vi "Check and Get Scalar.vi"(8 "error in (no error)":errorcluster, 9 "test commands":string[](array[string]), 10 "variable name":string, 11 "pipe in":T1) -> (0 "error out":errorcluster, 1 "variable":string, 2 "all tests OK?":bool, 3 "pipe out":T1)   [LabVIEW 2013, in "GOLPI library.lvlib"]
doc: "Checks scalar variable and gets it from GNU Octave in one write-read cycle. 'variable name' is the name of the variable. 'test commands' is array of GNU Octave commands with boolean output applied to the variable. I.e. to read noncomplex double scalar variable 'x', following array should be supplied:\nisnumeric\nisscalar\n~isscomplex\nTests performed are:\nisnumeric(x)\nisscalar(x)\n~iscomplex(x)\nIf output of all tests is '1', output 'all tests OK?' is true."
uses:
  GOLPI library.lvlib
  LV Process.lvlibp/Pipe Handle.ctl
  Utilities/Custom Error Codes Enum Type Def.vi
  Globals.vi
  LV Process.lvlibp
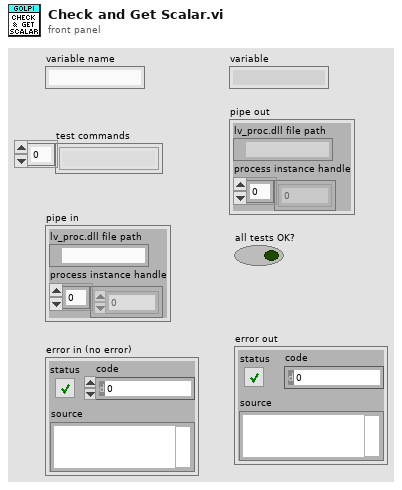
[diagram p1: front panel]
types:
  T1 = typedef "LV Process.lvlibp/Pipe Handle.ctl" = cluster{"lv_proc.dll file path":path, "process instance handle":u32[]}
  T2 = typedef "GOLPI library.lvlib/Custom Error Codes Enum Type Def.vi" = enum16{"no error", "00 working directory PAR1 missing", "01 octave binary PAR1 missing", "02 octave report error PAR1", "03 empty output last cmd PAR1", "04 missing temporary file PAR1", "10 var PAR1 not string", "11 var PAR1 not num, scal, ~compl", "12 var PAR1 not num, scal, compl", "13 var PAR1 not num, vect, ~compl", "14 var PAR1 not num, vect, compl", "15 var PAR1 not num, mat, ~compl", "16 var PAR1 not num, mat, ~compl", "99 not finished"}
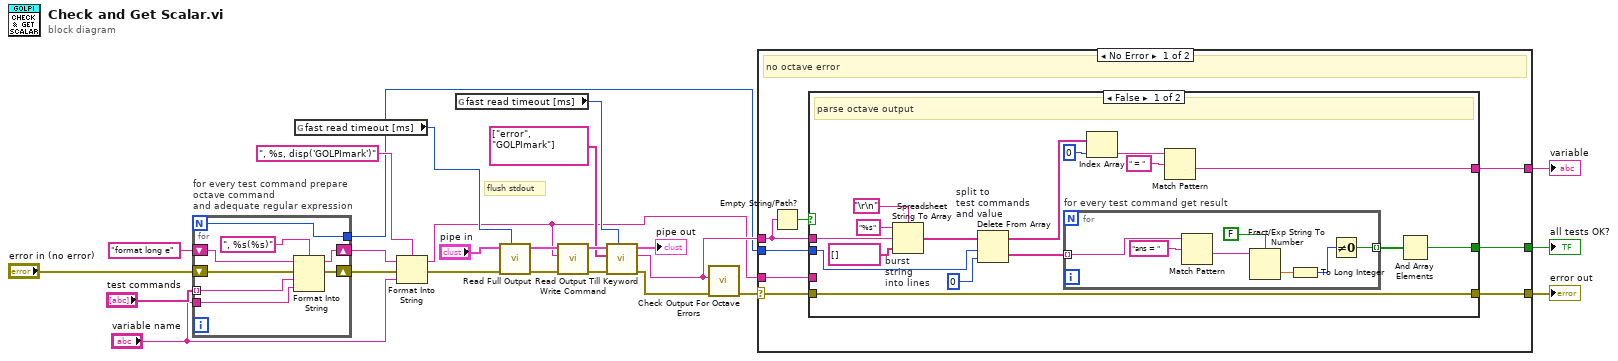
[diagram p0: block diagram]
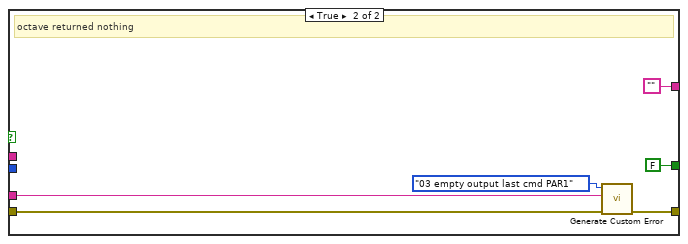
[diagram p2: hidden frame]
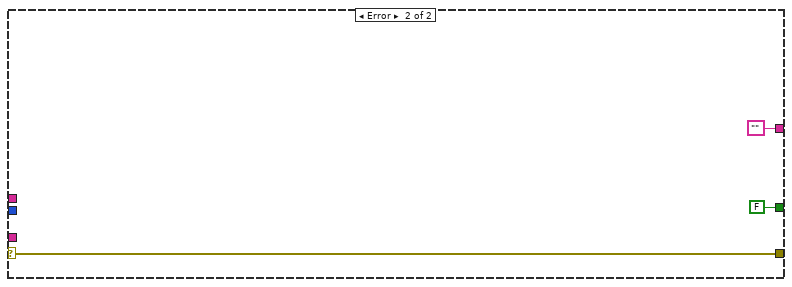
[diagram p3: hidden frame]
diagram:
  # "flush stdout"
  n1 = for "for every test command prepare\noctave command\nand adequate regular expression" {
    N -> [w26]
    tunnel: "test commands" -> [w31] mode=indexing
    tunnel: "variable name" -> [w30]
    shift-right: [w29] -> w2
    shift-left: "format long e" -> [w32]
    shift-right: [w27] -> w19
    shift-left: "error in (no error)" -> [w28]
    tunnel: [w26] -> w1
    n2 = Format Into String(format string=", %s(%s)", initial string=w32, error in=w28, w31, w30) -> (resulting string=w29:string, error out=w27:errorcluster)
  }
  n3 = global read "Globals.vi" "fast read timeout [ms]"() -> (w5:u32)
  n4 = Format Into String(format string=", %s, disp('GOLPImark')", initial string=w2, error in=w19, "variable name") -> (resulting string=w3:string, error out=w13:errorcluster)
  n5 = global read "Globals.vi" "fast read timeout [ms]"() -> (w12:u32)
  n6 = call "Read Full Output.vi"("timeout [ms]"=w5, "error in"=w13, "pipe in"="pipe in") -> ("error out"=w14:errorcluster, "pipe out"=w15:T1)  [unwired: 5 in, 2 out]
  n7 = call "Write Command.vi"("error in"=w14, "command"=w3, "pipe in"=w15) -> ("error out"=w11:errorcluster, "pipe out"=w7:T1)  [unwired: 7 in]
  n8 = call "Read Output Till Keyword.vi"("timeout [ms]"=w12, "error in"=w11, "keywords"=string[] ["error", "GOLPImark"], "pipe in"=w7) -> ("error out"=w10:errorcluster, "read buffer"=w9:string, "pipe out"=→"pipe out":T1)  [unwired: 4 in, 1 out]
  n9 = call "Check Output For Octave Errors.vi"("error in"=w10, "read buffer"=w9) -> ("error out"=w4:errorcluster)  [unwired: 9 in]
  n10 = case shown="No Error" w4 {
    selector: w4 -> [w37 w73]
    tunnel: [w41 ""] -> w21
    tunnel: [w40 FALSE] -> w20
    tunnel: [w39 w73] -> w18
    tunnel: w9 -> [w38 _]
    tunnel: w3 -> [w35 _]
    tunnel: w1 -> [w34 _]
    frame No Error {
      # "no octave error"
      n11 = Empty String/Path?(string/path=w38) -> (empty?=w36:bool)
      n12 = case shown="False" w36 {
        tunnel: [w42 ""] -> w41
        tunnel: [w50 FALSE] -> w40
        tunnel: [w49 w65] -> w39
        tunnel: w38 -> [w48 _]
        tunnel: w37 -> [w49 w66]
        tunnel: w35 -> [_ w67]
        tunnel: w34 -> [w47 _]
        frame False {
          # "parse octave output"
          n13 = Spreadsheet String To Array "burst\nstring\ninto lines"(delimiter (Tab)="\r\n", format string="%s", spreadsheet string=w48, array type (2D Dbl)=string[] []) -> (array=w54:string[])
          n14 = Delete From Array "split to\ntest commands\nand value"(array=w54, length=w47, index=0) -> (deleted portion=w56:string[], array with subset deleted=w45:string[])
          n15 = for "for every test command get result" {
            tunnel: w56 -> [w64] mode=indexing
            tunnel: [w58] -> w57 mode=indexing
            n16 = Match Pattern(string=w64, regular expression="ans = ") -> (after substring=w60:string)  [unwired: 1 in, 3 out]
            n17 = Fract/Exp String To Number(use system decimal point (T)=FALSE, string=w60) -> (number=w61:dbl)  [unwired: 2 in, 1 out]
            n18 = To Long Integer(number=w61) -> (32bit integer=w62:i32)
            n19 = Not Equal To 0?(x=w62) -> (x != 0?=w58:bool)
          }
          n20 = Index Array(array=w45, index=0) -> (element=w43:string)
          n21 = Match Pattern(string=w43, regular expression=" = ") -> (after substring=w42:string)  [unwired: 1 in, 3 out]
          n22 = And Array Elements(Boolean array=w57) -> (logical AND=w50:bool)
        }
        frame True {
          # "octave returned nothing"
          n23 = call "Generate Custom Error.vi"("error in"=w66, "PAR1"=w67, "GOLPI error"=Custom_Error_Codes_Enum_Type_Def.vi."03 empty output last cmd PAR1" ("Enum")) -> ("error out"=w65:errorcluster)  [unwired: 8 in]
        }
      }
    }
    frame Error {
    }
  }
  "all tests OK?" <- w20
  "variable" <- w21
  "error out" <- w18
